vi "initialize.vi"(0 "HGF_Agent":refnum<class "HB_PollingAgent.lvclass">, 3 "initializationData":variant, 5 "error in (no error)":errorcluster, 7 "binaryString":string, 8 "I8 Array":i8[](array[numeric]), 9 "prependSize? (T)":bool, 11 "byteOrder (0:big-endian, network order)":T1(ring)) -> (14 "dup HGF_Agent":refnum<class "HB_PollingAgent.lvclass">, 17 "found?":bool, 19 "error out":errorcluster)   [LabVIEW 2009, in "HB_PollingAgent.lvlib" / "HB_PollingAgent.lvclass"]
doc: "This is a dynamic dispatch VI to be implemented by child classes to initialize their attributes.\n\n<B>Recommendation:</B> Use Variant for initialization data."
uses:
  HB_PollingAgent.lvclass
  lib.lib/HGF_LVC/HGF_MobileAgentSystem/MoAgSy_AgentBase/MoAgSy_AgentBase.lvclass
  HB_PollingAgent.lvclass/HB_PollingAgent.ctl
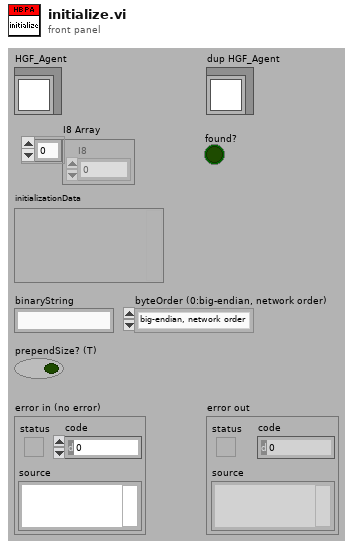
[diagram p1: front panel]
types:
  T1 = enum16{"big-endian, network order", "native, host order", "little-endian"}
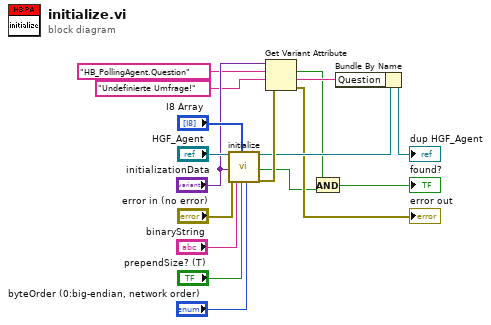
[diagram p0: block diagram]
diagram:
  n1 = call-parent "initialize.vi"("HGF_Agent"="HGF_Agent", "initializationData"="initializationData", "error in (no error)"="error in (no error)", "binaryString"="binaryString", "I8 Array"="I8 Array", "prependSize? (T)"="prependSize? (T)", "byteOrder (0:big-endian, network order)"="byteOrder (0:big-endian, network order)") -> ("dup HGF_Agent"=w9:refnum<class "HB_PollingAgent.lvclass">, "found?"=w3:bool, "error out"=w10:errorcluster)  [unwired: 10 in]
  n2 = Get Variant Attribute(Variant="initializationData", name="HB_PollingAgent.Question", default value (empty Variant)="Undefinierte Umfrage!", error in=w10) -> (found=w5:bool, value=w6:string, error out=→"error out":errorcluster)  [unwired: 1 out]
  n3 = And(x=w5, y=w3) -> (x .and. y?=→"found?":bool)
  n4 = Bundle By Name(cluster=w9, "Question"=w6) -> (→"dup HGF_Agent":refnum<class "HB_PollingAgent.lvclass">)
